vi "Project VI.vi"() -> ()   [LabVIEW 2022 SP3]
uses:
  <vilib>/DAQmx/read.llb/DAQmx Read (Digital Bool 1Line 1Point).vi
  <vilib>/DAQmx/write.llb/DAQmx Write (Digital Bool 1Line 1Point).vi
  <vilib>/DAQmx/read.llb/DAQmx Read (Analog DBL 1Chan 1Samp).vi
  <vilib>/DAQmx/create/channels.llb/DAQmx Create Channel (DI-Digital Input).vi
  <vilib>/DAQmx/create/channels.llb/DAQmx Create Channel (DO-Digital Output).vi
  <vilib>/DAQmx/create/channels.llb/DAQmx Create Channel (AI-Voltage-Basic).vi
  <vilib>/DAQmx/miscellaneous.llb/DAQmx Fill In Error Info.vi
panel:
  in  "?":tag
  out "?":bool
  out "Thermometer 2":dbl(slide) scale=25.0..60.0
  out "Waveform Chart 2":dbl(graph)
  out "Numeric 4":i32
  out "Numeric 3":i32
  out "Cleaning needed":bool
  out "LDR 05":bool
  in  "stop":bool
  in  "lines 10":tag
  in  "lines 9":tag
  in  "lines 8":tag
  in  "lines 7":tag
  in  "lines 6":tag
  in  "lines 5":tag
  out "LDR 04":bool
  in  "lines 4":tag
  out "LDR 03":bool
  in  "lines 3":tag
  out "LDR 02":bool
  in  "lines 2":tag
  out "LDR 01":bool
  in  "lines":tag
  # "LDR input"
  # "arduino OUT"
  # "TEMP Warning"
  # "Temp"
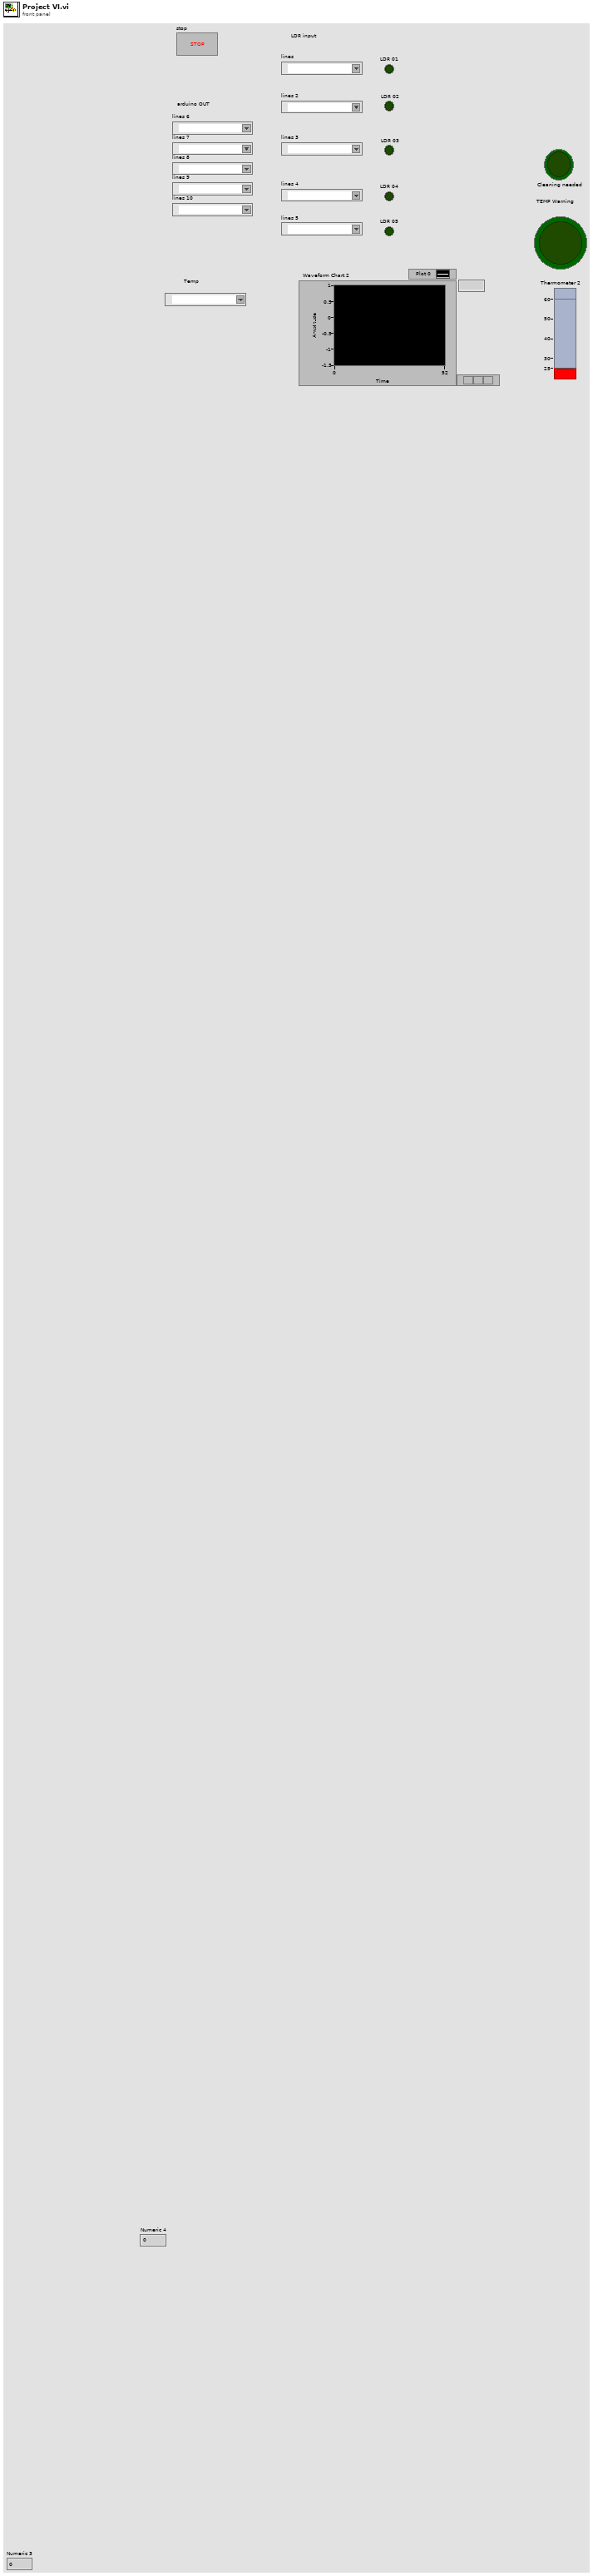
[diagram p1: front panel]
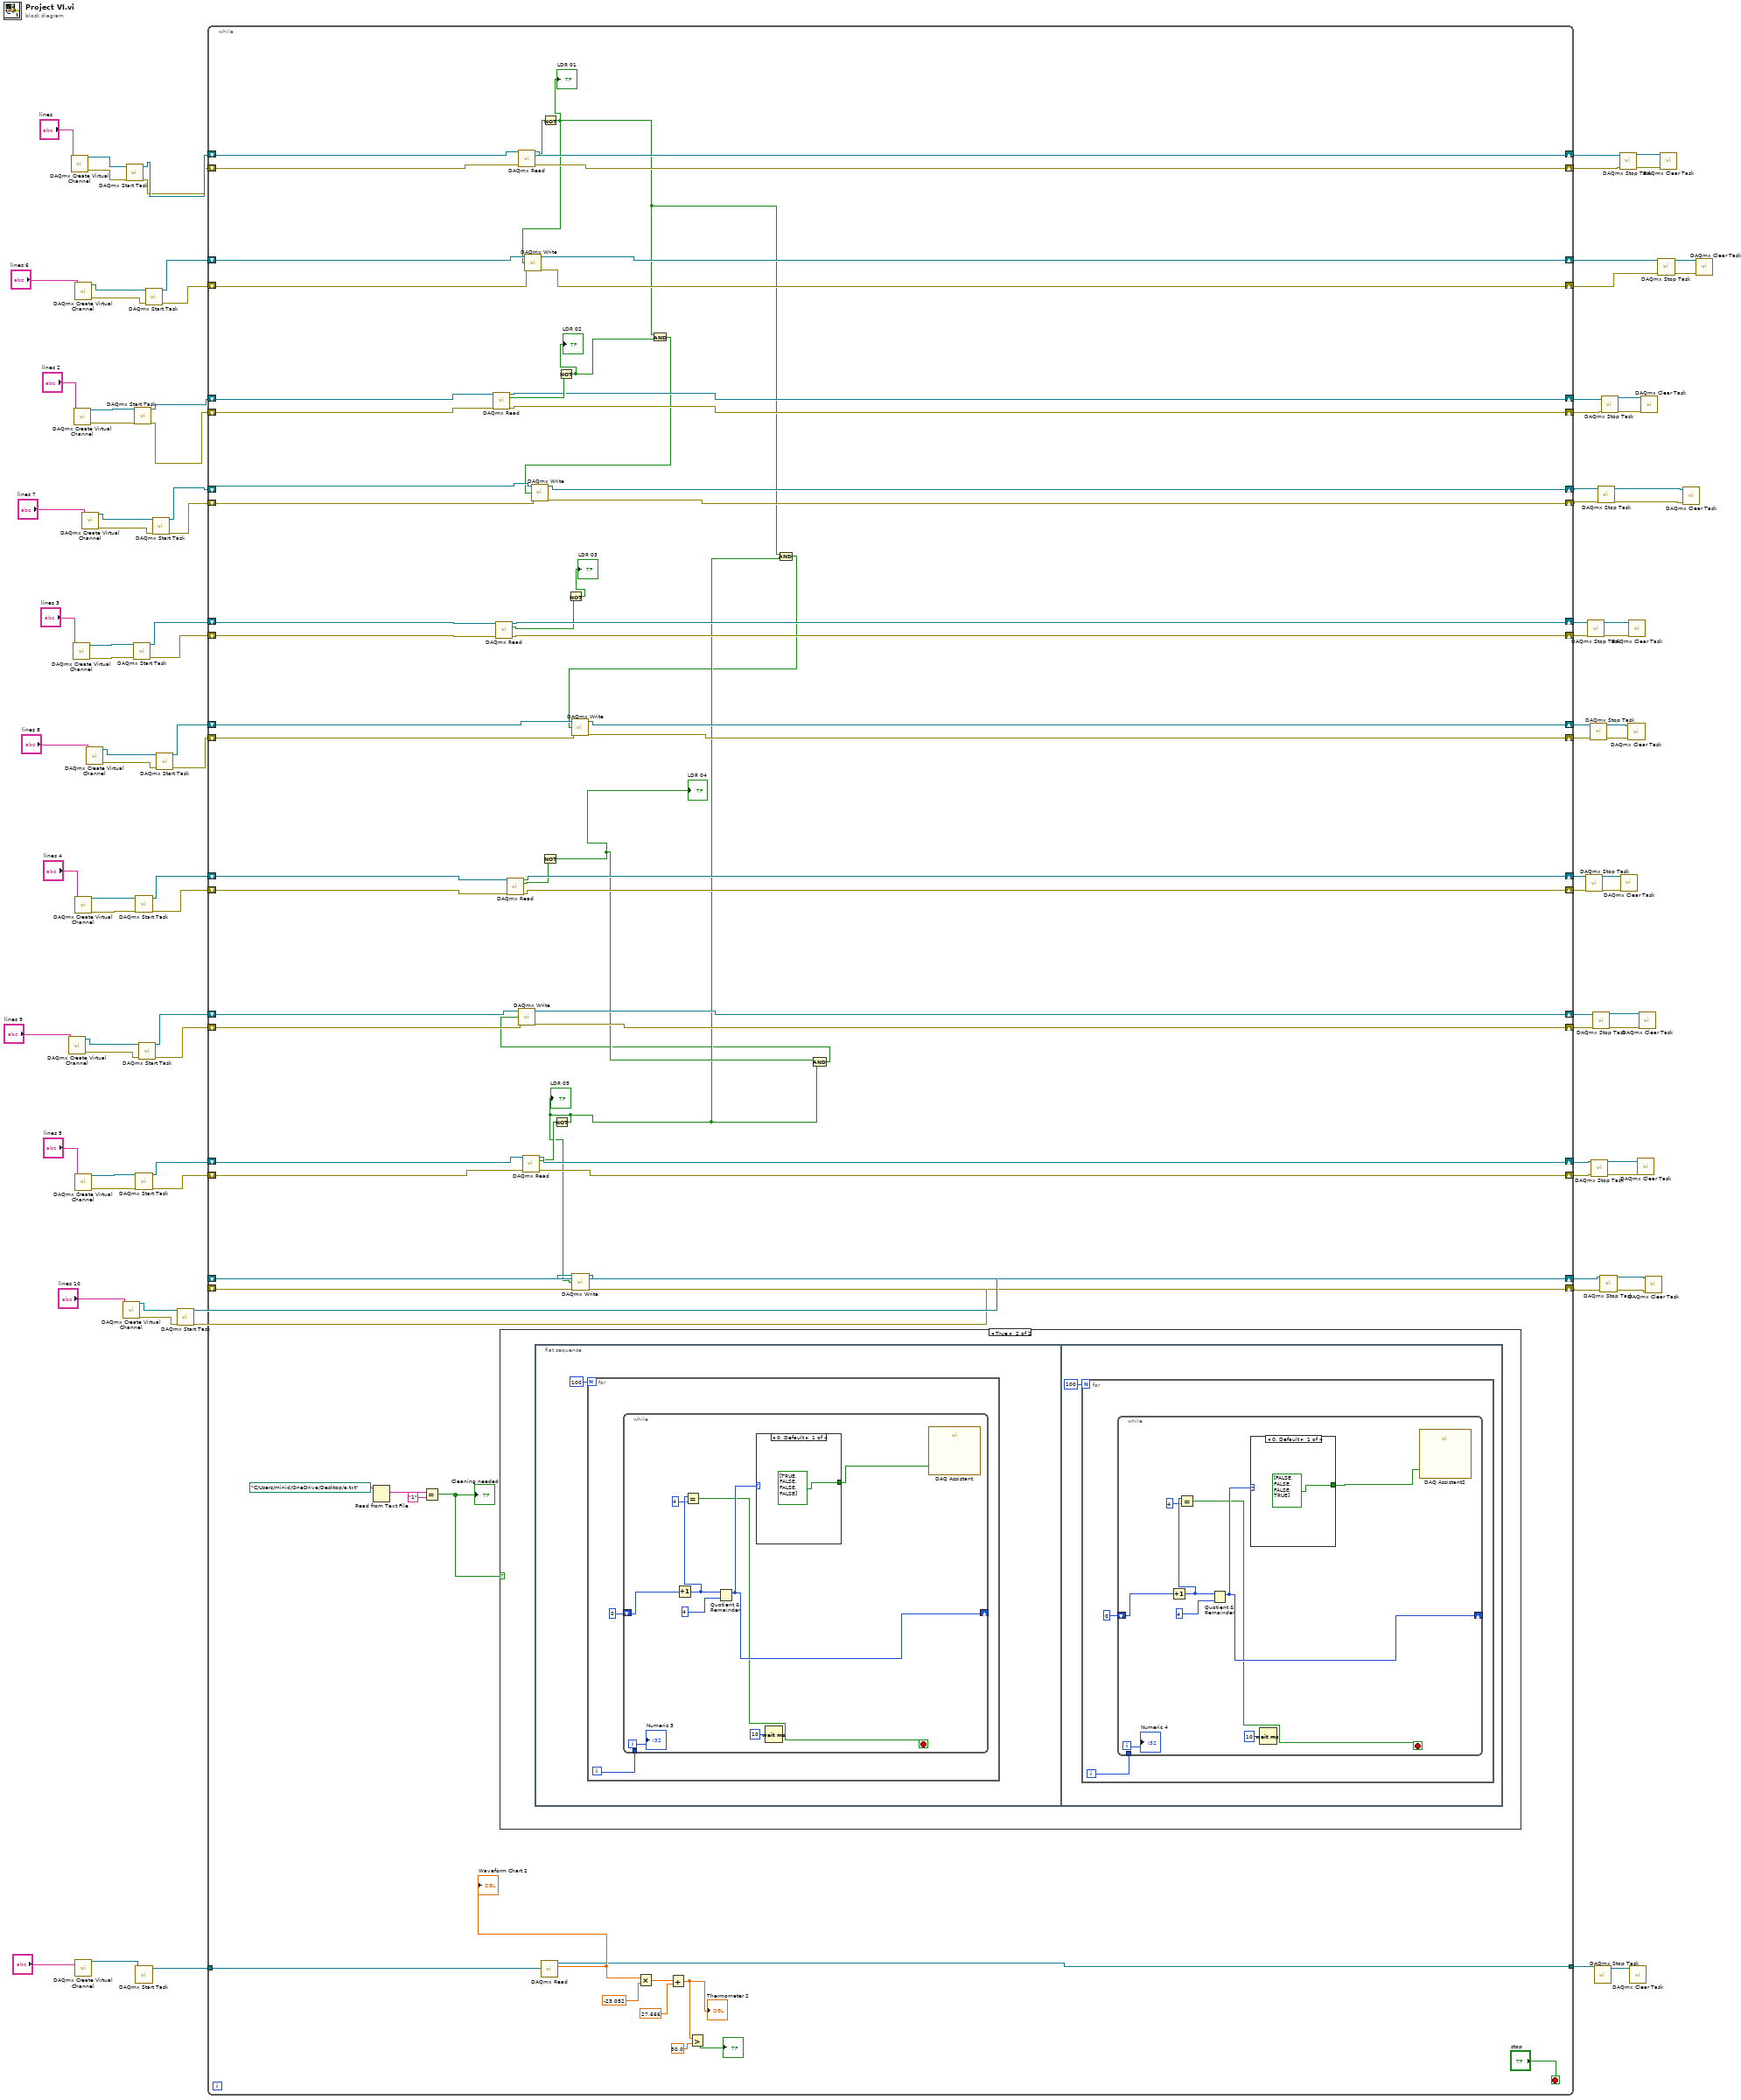
[diagram p0: block diagram]
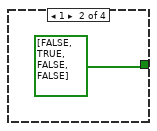
[diagram p3: hidden frame]
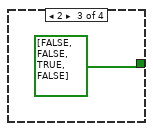
[diagram p4: hidden frame]
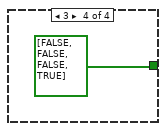
[diagram p5: hidden frame]
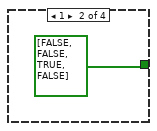
[diagram p6: hidden frame]
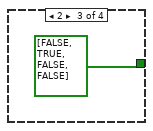
[diagram p7: hidden frame]
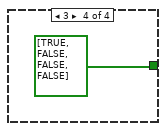
[diagram p8: hidden frame]
diagram:
  n1 = call-poly <vilib>:"DAQmx Create Virtual Channel.vi"("lines"="lines 9") -> ("task out"=w47:refnum<k21>, "error out"=w46:errorcluster)  [unwired: 13 in]
  n2 = call-poly <vilib>:"DAQmx Create Virtual Channel.vi"("lines"="lines") -> ("task out"=w95:refnum<k21>, "error out"=w92:errorcluster)  [unwired: 13 in]
  n3 = call-poly <vilib>:"DAQmx Create Virtual Channel.vi"("lines"="lines 3") -> ("task out"=w82:refnum<k21>, "error out"=w79:errorcluster)  [unwired: 13 in]
  n4 = call-poly <vilib>:"DAQmx Create Virtual Channel.vi"("lines"="lines 2") -> ("task out"=w87:refnum<k21>, "error out"=w85:errorcluster)  [unwired: 13 in]
  n5 = call-poly <vilib>:"DAQmx Create Virtual Channel.vi"("lines"="lines 6") -> ("task out"=w61:refnum<k21>, "error out"=w60:errorcluster)  [unwired: 13 in]
  n6 = call-poly <vilib>:"DAQmx Create Virtual Channel.vi"("lines"="lines 4") -> ("task out"=w75:refnum<k21>, "error out"=w72:errorcluster)  [unwired: 13 in]
  n7 = call-poly <vilib>:"DAQmx Create Virtual Channel.vi"("lines"="lines 5") -> ("task out"=w68:refnum<k21>, "error out"=w65:errorcluster)  [unwired: 13 in]
  n8 = call-poly <vilib>:"DAQmx Create Virtual Channel.vi"("physical channels"="?") -> ("task out"=w28:refnum<k21>)  [unwired: 13 in, 1 out]
  n9 = call-poly <vilib>:"DAQmx Create Virtual Channel.vi"("lines"="lines 7") -> ("task out"=w58:refnum<k21>, "error out"=w56:errorcluster)  [unwired: 13 in]
  n10 = call-poly <vilib>:"DAQmx Create Virtual Channel.vi"("lines"="lines 8") -> ("task out"=w53:refnum<k21>, "error out"=w50:errorcluster)  [unwired: 13 in]
  n11 = call-poly <vilib>:"DAQmx Create Virtual Channel.vi"("lines"="lines 10") -> ("task out"=w44:refnum<k21>, "error out"=w41:errorcluster)  [unwired: 13 in]
  n12 = call <vilib>:"DAQmx Start Task.vi"("task/channels in"=w95, "error in"=w92) -> ("task out"=w94:refnum<k21>, "error out"=w91:errorcluster)  [unwired: 12 in]
  n13 = call <vilib>:"DAQmx Start Task.vi"("task/channels in"=w82, "error in"=w79) -> ("task out"=w4:refnum<k21>, "error out"=w3:errorcluster)  [unwired: 12 in]
  n14 = call <vilib>:"DAQmx Start Task.vi"("task/channels in"=w87, "error in"=w85) -> ("task out"=w86:refnum<k21>, "error out"=w84:errorcluster)  [unwired: 12 in]
  n15 = call <vilib>:"DAQmx Start Task.vi"("task/channels in"=w75, "error in"=w72) -> ("task out"=w9:refnum<k21>, "error out"=w10:errorcluster)  [unwired: 12 in]
  n16 = call <vilib>:"DAQmx Start Task.vi"("task/channels in"=w68, "error in"=w65) -> ("task out"=w14:refnum<k21>, "error out"=w13:errorcluster)  [unwired: 12 in]
  n17 = call <vilib>:"DAQmx Start Task.vi"("task/channels in"=w28) -> ("task out"=w26:refnum<k21>)  [unwired: 13 in, 1 out]
  n18 = call <vilib>:"DAQmx Start Task.vi"("task/channels in"=w47, "error in"=w46) -> ("task out"=w12:refnum<k21>, "error out"=w11:errorcluster)  [unwired: 12 in]
  n19 = call <vilib>:"DAQmx Start Task.vi"("task/channels in"=w61, "error in"=w60) -> ("task out"=w8:refnum<k21>, "error out"=w7:errorcluster)  [unwired: 12 in]
  n20 = call <vilib>:"DAQmx Start Task.vi"("task/channels in"=w58, "error in"=w56) -> ("task out"=w6:refnum<k21>, "error out"=w5:errorcluster)  [unwired: 12 in]
  n21 = call <vilib>:"DAQmx Start Task.vi"("task/channels in"=w53, "error in"=w50) -> ("task out"=w2:refnum<k21>, "error out"=w1:errorcluster)  [unwired: 12 in]
  n22 = call <vilib>:"DAQmx Start Task.vi"("task/channels in"=w44, "error in"=w41) -> ("task out"=w43:refnum<k21>, "error out"=w40:errorcluster)  [unwired: 12 in]
  n23 = while {
    shift-right: [w161] -> w24
    shift-left: w94 -> [w162]
    shift-right: [w159] -> w90
    shift-left: w91 -> [w160]
    shift-right: [w119] -> w23
    shift-left: w86 -> [w158]
    shift-right: [w120] -> w29
    shift-left: w84 -> [w157]
    shift-right: [w155] -> w81
    shift-left: w4 -> [w156]
    shift-right: [w153] -> w78
    shift-left: w3 -> [w154]
    shift-right: [w151] -> w74
    shift-left: w9 -> [w152]
    shift-right: [w149] -> w71
    shift-left: w10 -> [w150]
    shift-right: [w147] -> w67
    shift-left: w14 -> [w148]
    shift-right: [w145] -> w64
    shift-left: w13 -> [w146]
    shift-right: [w122] -> w31
    shift-left: w8 -> [w139]
    shift-right: [w121] -> w30
    shift-left: w7 -> [w138]
    shift-right: [w137] -> w22
    shift-left: w6 -> [w124]
    shift-right: [w135] -> w21
    shift-left: w5 -> [w136]
    shift-right: [w133] -> w52
    shift-left: w2 -> [w134]
    shift-right: [w131] -> w49
    shift-left: w1 -> [w132]
    shift-right: [w118] -> w19
    shift-left: w12 -> [w130]
    shift-right: [w117] -> w18
    shift-left: w11 -> [w129]
    shift-right: [w127] -> w17
    shift-left: w43 -> [w128]
    shift-right: [w125] -> w16
    shift-left: w40 -> [w126]
    tunnel: w26 -> [w101]
    tunnel: [w100] -> w25
    stop <- "stop" stop-if-true
    n24 = Read from Text File(file (use dialog)=path "C:/Users/minid/OneDrive/Desktop/a.txt") -> (text=w112:string)  [unwired: 3 in, 3 out]
    n25 = Equal?(x=w112, y="1") -> (x = y?=w109:bool)
    "Cleaning needed" <- w109
    n26 = call-poly <vilib>:"DAQmx Read.vi"("task/channels in"=w158, "error in"=w157) -> ("task out"=w119:refnum<k21>, "data"=w143:bool, "error out"=w120:errorcluster)  [unwired: 11 in]
    n27 = call-poly <vilib>:"DAQmx Read.vi"("task/channels in"=w156, "error in"=w154) -> ("task out"=w155:refnum<k21>, "data"=w142:bool, "error out"=w153:errorcluster)  [unwired: 11 in]
    n28 = case shown="True" w109 {
      frame False {
      }
      frame True {
        n29 = flat-sequence {
          frame #0 {
            n30 = for {
              N: 100 -> [_]
              i -> [w164]
              n31 = while {
                shift-right: [w172] -> _
                shift-left: 0 -> [w174]
                tunnel: w164 -> [_]
                i -> [w170]
                stop <- w167 stop-if-true
                n32 = Increment(x=w174) -> (x+1=w169:i32)
                n33 = Equal?(x=w169, y=4) -> (x = y?=w167:bool)
                n34 = Quotient & Remainder(x=w169, y=4) -> (x-y*floor(x/y)=w172:i32)  [unwired: 1 out]
                n35 = case shown="0, Default" w172 {
                  tunnel: [bool[] [TRUE, FALSE, FALSE, FALSE] bool[] [FALSE, TRUE, FALSE, FALSE] bool[] [FALSE, FALSE, TRUE, FALSE] bool[] [FALSE, FALSE, FALSE, TRUE]] -> w166
                  frame 0, Default {
                  }
                  frame 1 {
                  }
                  frame 2 {
                  }
                  frame 3 {
                  }
                }
                n36 = Wait (ms)(milliseconds to wait=u32 10) -> ()  [unwired: 1 out]
                n37 = call "DAQ Assistant"("data"=w166) -> ()  [unwired: 17 in, 2 out]
                "Numeric 3" <- w170
              }
            }
          }
          frame #1 {
            n38 = for {
              N: 100 -> [_]
              i -> [w180]
              n39 = while {
                shift-right: [w188] -> _
                shift-left: 0 -> [w190]
                tunnel: w180 -> [_]
                i -> [w186]
                stop <- w183 stop-if-true
                n40 = Increment(x=w190) -> (x+1=w185:i32)
                n41 = Equal?(x=w185, y=4) -> (x = y?=w183:bool)
                n42 = Quotient & Remainder(x=w185, y=4) -> (x-y*floor(x/y)=w188:i32)  [unwired: 1 out]
                n43 = case shown="0, Default" w188 {
                  tunnel: [bool[] [FALSE, FALSE, FALSE, TRUE] bool[] [FALSE, FALSE, TRUE, FALSE] bool[] [FALSE, TRUE, FALSE, FALSE] bool[] [TRUE, FALSE, FALSE, FALSE]] -> w182
                  frame 0, Default {
                  }
                  frame 1 {
                  }
                  frame 2 {
                  }
                  frame 3 {
                  }
                }
                n44 = Wait (ms)(milliseconds to wait=u32 10) -> ()  [unwired: 1 out]
                n45 = call "DAQ Assistant2"("data"=w182) -> ()  [unwired: 17 in, 2 out]
                "Numeric 4" <- w186
              }
            }
          }
        }
      }
    }
    n46 = call-poly <vilib>:"DAQmx Read.vi"("task/channels in"=w152, "error in"=w150) -> ("task out"=w151:refnum<k21>, "data"=w141:bool, "error out"=w149:errorcluster)  [unwired: 11 in]
    n47 = call-poly <vilib>:"DAQmx Read.vi"("task/channels in"=w162, "error in"=w160) -> ("task out"=w161:refnum<k21>, "data"=w144:bool, "error out"=w159:errorcluster)  [unwired: 11 in]
    n48 = call-poly <vilib>:"DAQmx Read.vi"("task/channels in"=w148, "error in"=w146) -> ("task out"=w147:refnum<k21>, "data"=w140:bool, "error out"=w145:errorcluster)  [unwired: 11 in]
    n49 = call-poly <vilib>:"DAQmx Read.vi"("task/channels in"=w101) -> ("task out"=w100:refnum<k21>, "data"=w107:dbl)  [unwired: 12 in, 1 out]
    "Waveform Chart 2" <- w107
    n50 = Not(x=w141) -> (.not. x?=w114:bool)
    "LDR 04" <- w114
    n51 = Not(x=w144) -> (.not. x?=w99:bool)
    "LDR 01" <- w99
    n52 = call-poly <vilib>:"DAQmx Write.vi"("task/channels in"=w139, "data"=w99, "error in"=w138) -> ("task out"=w122:refnum<k21>, "error out"=w121:errorcluster)  [unwired: 10 in, 1 out]
    n53 = Not(x=w140) -> (.not. x?=w98:bool)
    "LDR 05" <- w98
    n54 = Not(x=w143) -> (.not. x?=w116:bool)
    "LDR 02" <- w116
    n55 = Not(x=w142) -> (.not. x?=→"LDR 03":bool)
    n56 = call-poly <vilib>:"DAQmx Write.vi"("task/channels in"=w128, "data"=w98, "error in"=w126) -> ("task out"=w127:refnum<k21>, "error out"=w125:errorcluster)  [unwired: 10 in, 1 out]
    n57 = Multiply(x=w107, y=-23.052) -> (x*y=w106:dbl)
    n58 = And(x=w99, y=w116) -> (x .and. y?=w115:bool)
    n59 = call-poly <vilib>:"DAQmx Write.vi"("task/channels in"=w124, "data"=w115, "error in"=w136) -> ("task out"=w137:refnum<k21>, "error out"=w135:errorcluster)  [unwired: 10 in, 1 out]
    n60 = Add(x=w106, y=27.666) -> (x+y=w104:dbl)
    "Thermometer 2" <- w104
    n61 = Greater?(x=w104, y=50.0) -> (0:→"?":bool)
    n62 = And(x=w99, y=w98) -> (x .and. y?=w96:bool)
    n63 = call-poly <vilib>:"DAQmx Write.vi"("task/channels in"=w134, "data"=w96, "error in"=w132) -> ("task out"=w133:refnum<k21>, "error out"=w131:errorcluster)  [unwired: 10 in, 1 out]
    n64 = And(x=w114, y=w98) -> (x .and. y?=w97:bool)
    n65 = call-poly <vilib>:"DAQmx Write.vi"("task/channels in"=w130, "data"=w97, "error in"=w129) -> ("task out"=w118:refnum<k21>, "error out"=w117:errorcluster)  [unwired: 10 in, 1 out]
  }
  n66 = call <vilib>:"DAQmx Stop Task.vi"("task/channels in"=w74, "error in"=w71) -> ("task out"=w73:refnum<k21>, "error out"=w70:errorcluster)  [unwired: 12 in]
  n67 = call <vilib>:"DAQmx Stop Task.vi"("task/channels in"=w81, "error in"=w78) -> ("task out"=w80:refnum<k21>, "error out"=w77:errorcluster)  [unwired: 12 in]
  n68 = call <vilib>:"DAQmx Stop Task.vi"("task/channels in"=w52, "error in"=w49) -> ("task out"=w51:refnum<k21>, "error out"=w20:errorcluster)  [unwired: 12 in]
  n69 = call <vilib>:"DAQmx Stop Task.vi"("task/channels in"=w67, "error in"=w64) -> ("task out"=w66:refnum<k21>, "error out"=w63:errorcluster)  [unwired: 12 in]
  n70 = call <vilib>:"DAQmx Stop Task.vi"("task/channels in"=w19, "error in"=w18) -> ("task out"=w37:refnum<k21>, "error out"=w36:errorcluster)  [unwired: 12 in]
  n71 = call <vilib>:"DAQmx Stop Task.vi"("task/channels in"=w25) -> ("task out"=w15:refnum<k21>)  [unwired: 13 in, 1 out]
  n72 = call <vilib>:"DAQmx Stop Task.vi"("task/channels in"=w22, "error in"=w21) -> ("task out"=w57:refnum<k21>, "error out"=w55:errorcluster)  [unwired: 12 in]
  n73 = call <vilib>:"DAQmx Stop Task.vi"("task/channels in"=w17, "error in"=w16) -> ("task out"=w42:refnum<k21>, "error out"=w39:errorcluster)  [unwired: 12 in]
  n74 = call <vilib>:"DAQmx Stop Task.vi"("task/channels in"=w23, "error in"=w29) -> ("task out"=w35:refnum<k21>, "error out"=w34:errorcluster)  [unwired: 12 in]
  n75 = call <vilib>:"DAQmx Stop Task.vi"("task/channels in"=w24, "error in"=w90) -> ("task out"=w93:refnum<k21>, "error out"=w89:errorcluster)  [unwired: 12 in]
  n76 = call <vilib>:"DAQmx Clear Task.vi"("task in"=w73, "error in"=w70) -> ()  [unwired: 13 in, 1 out]
  n77 = call <vilib>:"DAQmx Clear Task.vi"("task in"=w51, "error in"=w20) -> ()  [unwired: 13 in, 1 out]
  n78 = call <vilib>:"DAQmx Clear Task.vi"("task in"=w80, "error in"=w77) -> ()  [unwired: 13 in, 1 out]
  n79 = call <vilib>:"DAQmx Clear Task.vi"("task in"=w15) -> ()  [unwired: 14 in, 1 out]
  n80 = call <vilib>:"DAQmx Clear Task.vi"("task in"=w66, "error in"=w63) -> ()  [unwired: 13 in, 1 out]
  n81 = call <vilib>:"DAQmx Clear Task.vi"("task in"=w37, "error in"=w36) -> ()  [unwired: 13 in, 1 out]
  n82 = call <vilib>:"DAQmx Clear Task.vi"("task in"=w35, "error in"=w34) -> ()  [unwired: 13 in, 1 out]
  n83 = call <vilib>:"DAQmx Clear Task.vi"("task in"=w42, "error in"=w39) -> ()  [unwired: 13 in, 1 out]
  n84 = call <vilib>:"DAQmx Stop Task.vi"("task/channels in"=w31, "error in"=w30) -> ("task out"=w33:refnum<k21>, "error out"=w32:errorcluster)  [unwired: 12 in]
  n85 = call <vilib>:"DAQmx Clear Task.vi"("task in"=w93, "error in"=w89) -> ()  [unwired: 13 in, 1 out]
  n86 = call <vilib>:"DAQmx Clear Task.vi"("task in"=w57, "error in"=w55) -> ()  [unwired: 13 in, 1 out]
  n87 = call <vilib>:"DAQmx Clear Task.vi"("task in"=w33, "error in"=w32) -> ()  [unwired: 13 in, 1 out]
